vi "subTiE_GetStatus.vi"(1 "Ref":T2) -> (0 "TI-Ctrl":T1={"Obj"=1, "Cube 1"=0, "Cube 2"=1, "PFS-Ctrl"={"PFS IO"=FALSE, "PSF Err"=FALSE, "PSF Pos"=0}, "Z-Ctrl"={"Z-pos"=0.0, "Home"=FALSE, "Sensitivity"=1}, "Condenser"=1, "Lightpath"=enum."EYE"} {"Condenser" items=["- empty 1 -"=1, "- empty 2 -"=2, "- empty 3 -"=3, "- empty 4 -"=4, "- empty 5 -"=5, "- empty 6 -"=6]; "Z-Ctrl"."Sensitivity" min=1 max=3 step=1 scale=1.0..3.0; "PFS-Ctrl"."PSF Pos" scale=0.0..16400.0; "Cube 2" items=["- empty 1 -"=1, "- empty 2 -"=2, "- empty 3 -"=3, "- empty 4 -"=4, "- empty 5 -"=5, "- empty 6 -"=6]; "Cube 1" items=["DAPI"=1, "GFP"=2, "RHOD"=3, "Cy5"=4, "Trans"=5, "- empty 6 -"=6]; "Obj" items=["10x/0.3"=1, "- empty 2 -"=2, "- empty 3 -"=3, "100x/1.49 Oil"=4, "- empty 5 -"=5, "Aligner"=6]})   [LabVIEW 2015]
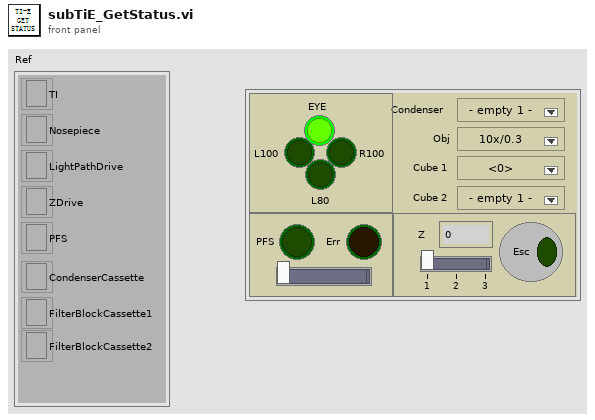
[diagram p1: front panel]
types:
  T1 = cluster{"Obj":u16, "Cube 1":u16, "Cube 2":u16, "PFS-Ctrl":cluster{"PFS IO":bool, "PSF Err":bool, "PSF Pos":u32}, "Z-Ctrl":cluster{"Z-pos":dbl, "Home":bool, "Sensitivity":u8}, "Condenser":u16, "Lightpath":enum32{"EYE", "L100", "R100", "L80"}}
  T2 = cluster{"TI":refnum<k7>, "Nosepiece":refnum<k7>, "LightPathDrive":refnum<k7>, "ZDrive":refnum<k7>, "PFS":refnum<k7>, "CondenserCassette":refnum<k7>, "FilterBlockCassette1":refnum<k7>, "FilterBlockCassette2":refnum<k7>}
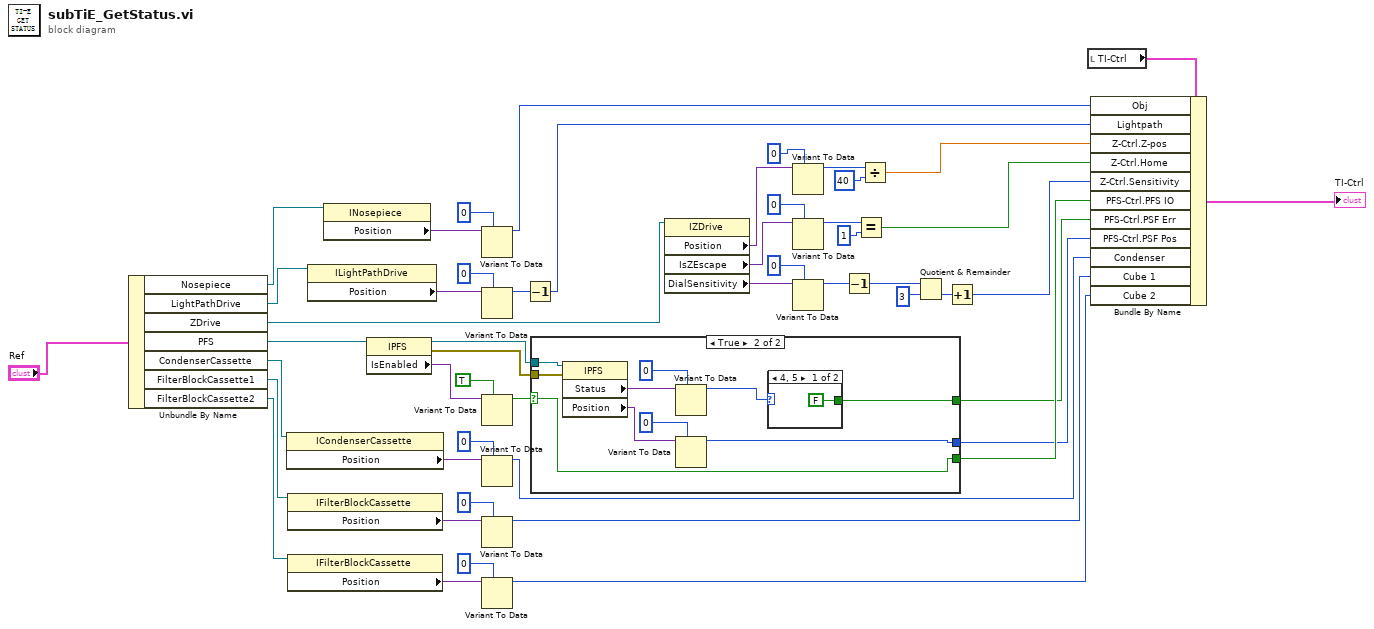
[diagram p0: block diagram]
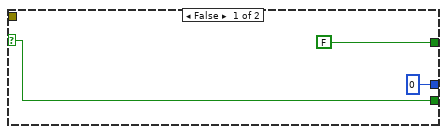
[diagram p2: hidden frame]
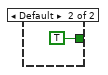
[diagram p3: hidden frame]
diagram:
  n1 = Unbundle By Name("Ref") -> ("Nosepiece"=w49:refnum<k7>, "LightPathDrive"=w18:refnum<k7>, "ZDrive"=w17:refnum<k7>, "PFS"=w16:refnum<k7>, "CondenserCassette"=w15:refnum<k7>, "FilterBlockCassette1"=w14:refnum<k7>, "FilterBlockCassette2"=w13:refnum<k7>)
  n2 = property class="ICondenserCassette"(reference=w15) -> ("Position"=w24:variant)  [unwired: 1 in, 2 out]
  n3 = property class="IFilterBlockCassette"(reference=w14) -> ("Position"=w22:variant)  [unwired: 1 in, 2 out]
  n4 = property class="IFilterBlockCassette"(reference=w13) -> ("Position"=w20:variant)  [unwired: 1 in, 2 out]
  n5 = property class="ILightPathDrive"(reference=w18) -> ("Position"=w45:variant)  [unwired: 1 in, 2 out]
  n6 = property class="INosepiece"(reference=w49) -> ("Position"=w48:variant)  [unwired: 1 in, 2 out]
  n7 = property class="IPFS"(reference=w16) -> (reference out=w27:refnum<k7>, error out=w26:errorcluster, "IsEnabled"=w29:variant)  [unwired: 1 in]
  n8 = Variant To Data(type=u16 0, Variant=w48) -> (data=w51:u16)  [unwired: 1 in, 1 out]
  n9 = Variant To Data(type=u16 0, Variant=w45) -> (data=w46:u16)  [unwired: 1 in, 1 out]
  n10 = Variant To Data(type=TRUE, Variant=w29) -> (data=w25:bool)  [unwired: 1 in, 1 out]
  n11 = Variant To Data(type=u16 0, Variant=w24) -> (data=w5:u16)  [unwired: 1 in, 1 out]
  n12 = Variant To Data(type=u16 0, Variant=w22) -> (data=w4:u16)  [unwired: 1 in, 1 out]
  n13 = Variant To Data(type=u16 0, Variant=w20) -> (data=w3:u16)  [unwired: 1 in, 1 out]
  n14 = Decrement(x=w46) -> (x-1=w12:u16)
  n15 = case shown="True" w25 {
    selector: w25 -> [w53 w55]
    tunnel: w26 -> [_ w64]
    tunnel: w27 -> [_ w63]
    tunnel: [u16 0 w61] -> w6
    tunnel: [FALSE w56] -> w7
    tunnel: [w53 w55] -> w8
    frame False {
    }
    frame True {
      n16 = property class="IPFS"(reference=w63, error in=w64) -> ("Status"=w58:variant, "Position"=w60:variant)  [unwired: 2 out]
      n17 = Variant To Data(type=u16 0, Variant=w58) -> (data=w57:u16)  [unwired: 1 in, 1 out]
      n18 = Variant To Data(type=u16 0, Variant=w60) -> (data=w61:u16)  [unwired: 1 in, 1 out]
      n19 = case shown="4, 5" w57 {
        tunnel: [FALSE TRUE] -> w56
        frame 4, 5 {
        }
        frame Default {
        }
      }
    }
  }
  n20 = property class="IZDrive"(reference=w17) -> ("Position"=w42:variant, "IsZEscape"=w40:variant, "DialSensitivity"=w38:variant)  [unwired: 1 in, 2 out]
  n21 = Variant To Data(type=u64 0, Variant=w42) -> (data=w37:u64)  [unwired: 1 in, 1 out]
  n22 = Variant To Data(type=0, Variant=w40) -> (data=w35:i32)  [unwired: 1 in, 1 out]
  n23 = Variant To Data(type=0, Variant=w38) -> (data=w33:i32)  [unwired: 1 in, 1 out]
  n24 = Decrement(x=w33) -> (x-1=w30:i32)
  n25 = Equal?(x=w35, y=1) -> (x = y?=w10:bool)
  n26 = Divide(x=w37, y=u64 40) -> (x/y=w11:dbl)
  n27 = Quotient & Remainder(x=w30, y=3) -> (floor(x/y)=w31:i32)  [unwired: 1 out]
  n28 = Increment(x=w31) -> (x+1=w9:i32)
  n29 = local read "TI-Ctrl"() -> (w50:T1)
  n30 = Bundle By Name(cluster=w50, "Obj"=w51, "Lightpath"=w12, "Z-Ctrl.Z-pos"=w11, "Z-Ctrl.Home"=w10, "Z-Ctrl.Sensitivity"=w9, "PFS-Ctrl.PFS IO"=w8, "PFS-Ctrl.PSF Err"=w7, "PFS-Ctrl.PSF Pos"=w6, "Condenser"=w5, "Cube 1"=w4, "Cube 2"=w3) -> (→"TI-Ctrl":T1)
